vi "agilent_test.vi"() -> ()   [LabVIEW 2016]
uses:
  <vilib>/Instr/_visa.llb/VISA Open Access Mode.ctl
  <vilib>/regexp/Match Regular Expression.xnode
panel:
  out "error out":errorcluster
  out "VISA resource name out":refnum<visa-resource-name>
  in  "ID Query (True)":bool=TRUE
  in  "VISA resource name":refnum<visa-resource-name>="vna"
  in  "error in (no error)":errorcluster
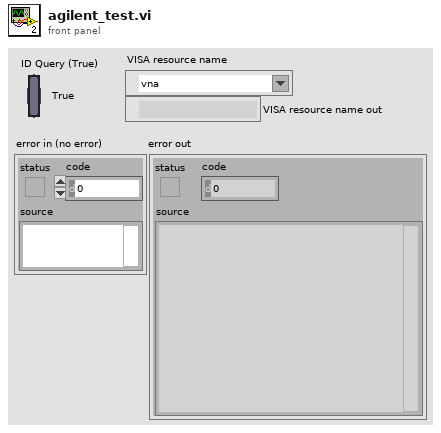
[diagram p1: front panel]
types:
  T1 = typedef "VISA Open Access Mode.ctl" = u32
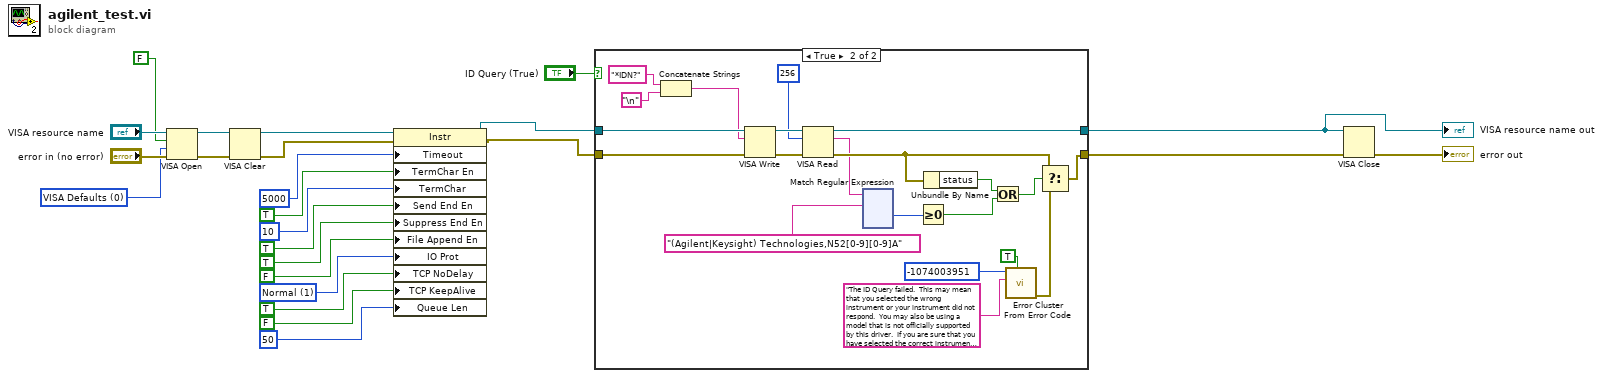
[diagram p0: block diagram]
diagram:
  w5 = T1 0 items=["VISA Defaults"=0, "Exclusive Lock"=1, "Load Configured Settings"=4] ("Access Mode")
  w12 = u16 1 items=["Normal"=1, "VXI/FDC"=2, "GPIB/HS488"=3, "Serial-TCPIP-USB/488 Strings"=4, "USBTMC/Vendor-Specific"=5] ("Message Based Settings:IO Protocol")
  n1 = VISA Open(duplicate session (F)=FALSE, access mode=w5, error in (no error)="error in (no error)", VISA resource name="VISA resource name") -> (VISA resource name=w22:refnum<visa-resource-name>, error out=w21:errorcluster)  [unwired: 1 in]
  n2 = VISA Clear(VISA resource name=w22, error in (no error)=w21) -> (VISA resource name out=w20:refnum<visa-resource-name>, error out=w19:errorcluster)
  n3 = property class="Instr"(reference=w20, error in=w19, "Timeout"=u32 5000 ("General Settings:Timeout Value"), "TermChar En"=TRUE ("Message Based Settings:Termination Character Enable"), "TermChar"=u8 10 ("Message Based Settings:Termination Character"), "Send End En"=TRUE ("Message Based Settings:Send End Enable"), "Suppress End En"=TRUE ("Message Based Settings:Suppress End Enable"), "File Append En"=FALSE ("Message Based Settings:File Append Enable"), "IO Prot"=w12, "TCP NoDelay"=TRUE ("TCP/IP Settings:No Packet Delay"), "TCP KeepAlive"=FALSE ("TCP/IP Settings:Keep-Alive Packets"), "Queue Len"=u32 50 ("General Settings:Maximum Queue Length")) -> (reference out=w7:refnum<visa-resource-name>, error out=w8:errorcluster)
  n4 = case shown="True" "ID Query (True)" {
    tunnel: [w25 w47] -> w3
    tunnel: [w26 w44] -> w2
    tunnel: w7 -> [w26 w45]
    tunnel: w8 -> [w25 w46]
    frame False {
    }
    frame True {
      n5 = Concatenate Strings("*IDN?" ("string"), "\n") -> (w27:string)
      n6 = VISA Write(VISA resource name=w45, write buffer=w27, error in (no error)=w46) -> (VISA resource name out=w43:refnum<visa-resource-name>, error out=w42:errorcluster)  [unwired: 1 out]
      n7 = VISA Read(VISA resource name=w43, byte count=u32 256, error in (no error)=w42) -> (VISA resource name out=w44:refnum<visa-resource-name>, read buffer=w30:string, error out=w36:errorcluster)  [unwired: 1 out]
      n8 = xnode "Match Regular Expression"("input string"=w30, "regular expression"="(Agilent|Keysight) Technologies,N52[0-9][0-9]A") -> ("offset past match"=w31:i32)  [unwired: 4 in, 4 out]
      n9 = Greater Or Equal To 0?(x=w31) -> (x >= 0?=w34:bool)
      n10 = Unbundle By Name(w36) -> ("status"=w35:bool)
      n11 = Or(x=w35, y=w34) -> (x .or. y?=w33:bool)
      n12 = call <vilib>:"Error Cluster From Error Code.vi"("show call chain? (False)"=TRUE, "error message (\"\")"="The ID Query failed.  This may mean that you selected the wrong instrument or your instrument did not respond.  You may also be using a model that is not officially supported by this driver.  If you are sure that you have selected the correct instrument and it is responding, try disabling the ID Query." ("Source (VI Name)"), "error code (0)"=-1074003951 ("Code")) -> ("error out"=w40:errorcluster)  [unwired: 6 in]
      n13 = Select(t=w36, s=w33, f=w40) -> (s? t:f=w47:errorcluster)
    }
  }
  "VISA resource name out" <- w2
  n14 = VISA Close(VISA resource name=w2, error in (no error)=w3) -> (error out=→"error out":errorcluster)
